vi "4-Build Do.vi"() -> ()   [LabVIEW 2014, in "TestVIs.lvlib"]
uses:
  TestVIs.lvlib
  <vilib>/Utility/traverseref.llb/TRef TravTarget.ctl
  <vilib>/Utility/miscctls.llb/LVPointTypeDef.ctl
  <vilib>/Utility/traverseref.llb/VI Scripting - Traverse.lvlib
  CSPP_Actor/CS++Actor.lvclass
panel:
  out "error out":errorcluster
  in  "error in (no error)":errorcluster
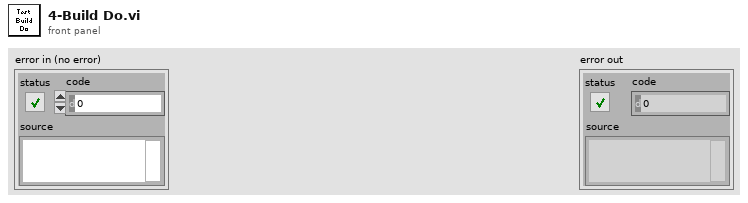
[diagram p1: front panel]
types:
  T1 = cluster{"Actor Method VI":refnum<vi>, "Actor Class":refnum<vi>, "Message Class":refnum<vi>}
  T2 = enum16{"Replace Class Controls/Constants", "Wire Special Inputs", "Wire Outputs", "Wire Method Inputs", "Connect Unbundler Input"}
  T3 = cluster{"Actor":cluster{"In":i32, "Out":i32}, "Error":cluster{"In":i32, "Out":i32}, "Terminals":cluster{"Position":enum16{"Left", "Top", "Bottom", "Right"}, "Terminal":i32}[]}
  T4 = typedef "TRef TravTarget.ctl" = enum16{"FP", "BD", "Other"}
  T5 = typedef "LVPointTypeDef.ctl" = cluster{"Horizontal":i16, "Vertical":i16}
  T6 = cluster{"Position":enum16{"Left", "Top", "Bottom", "Right"}, "Terminal":i32}[]
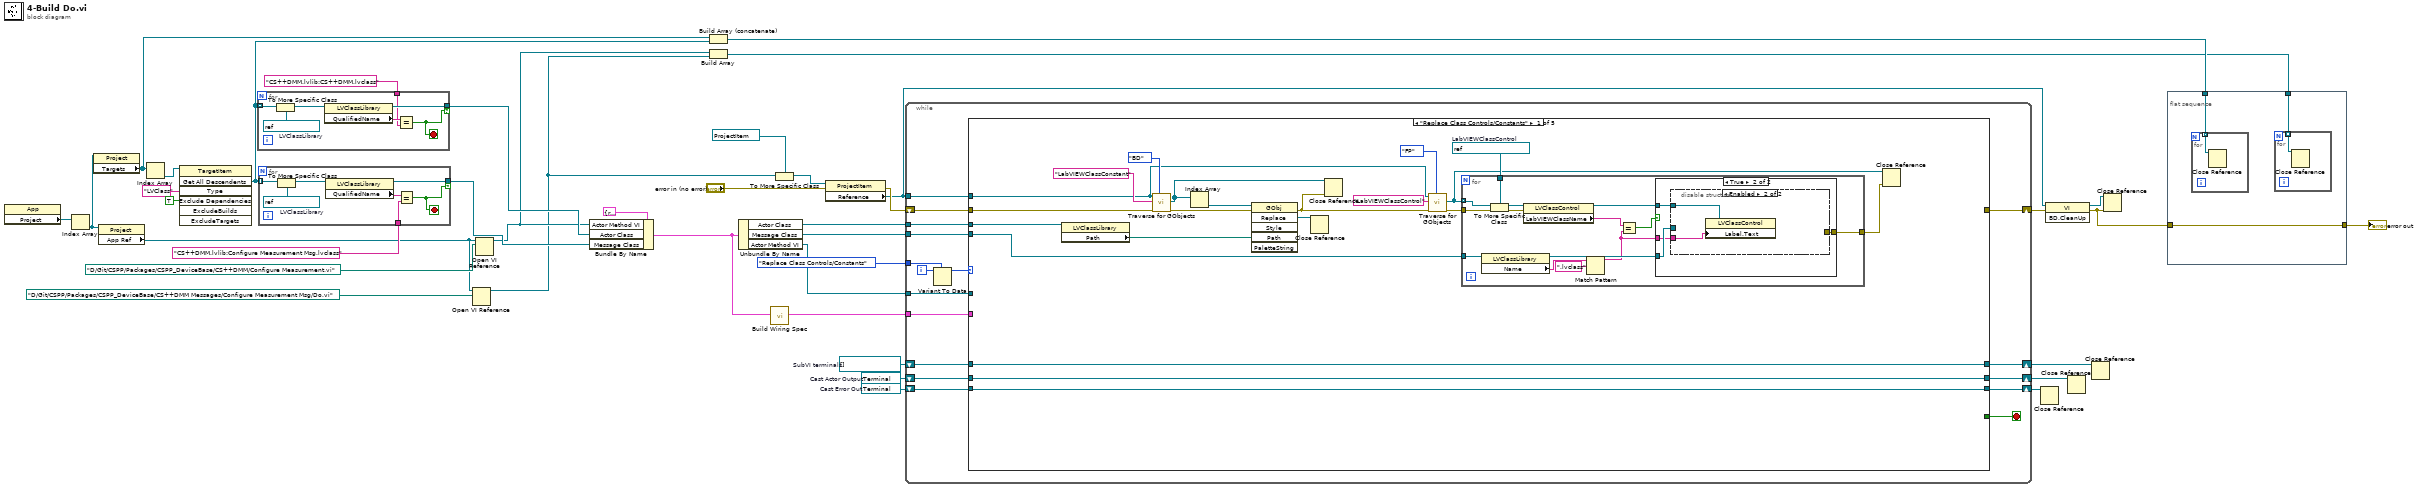
[diagram p0: block diagram]
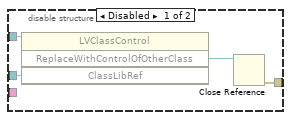
[diagram p3: hidden frame]
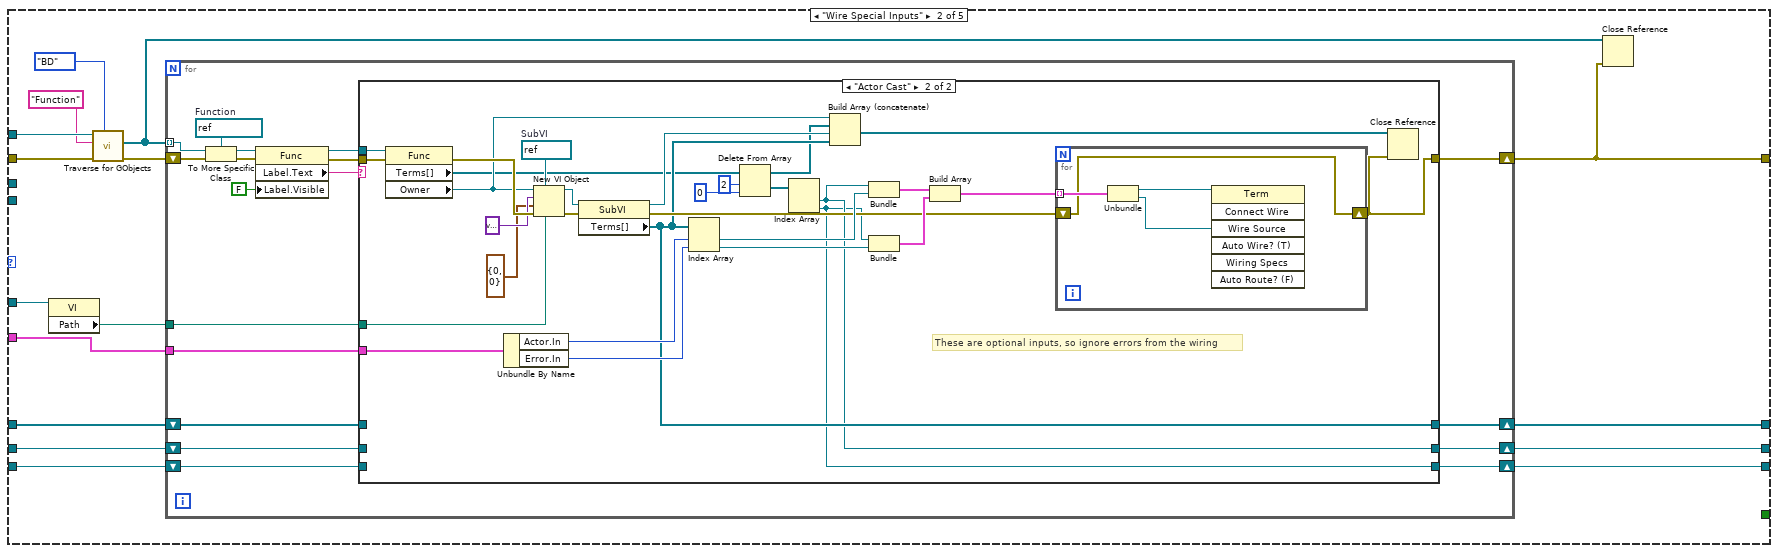
[diagram p4: hidden frame]
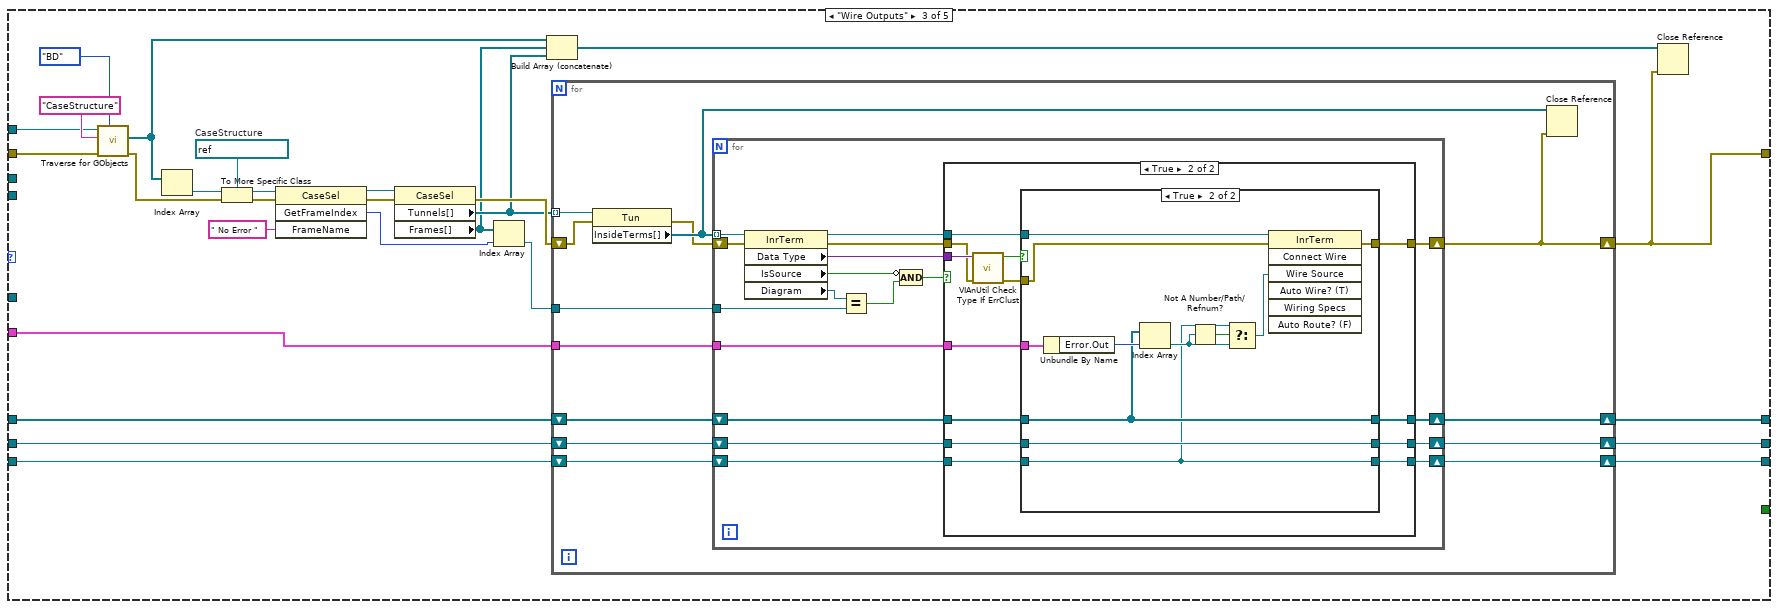
[diagram p6: hidden frame]
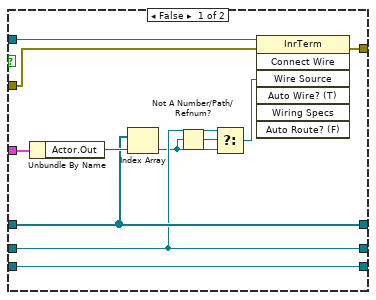
[diagram p8: hidden frame]
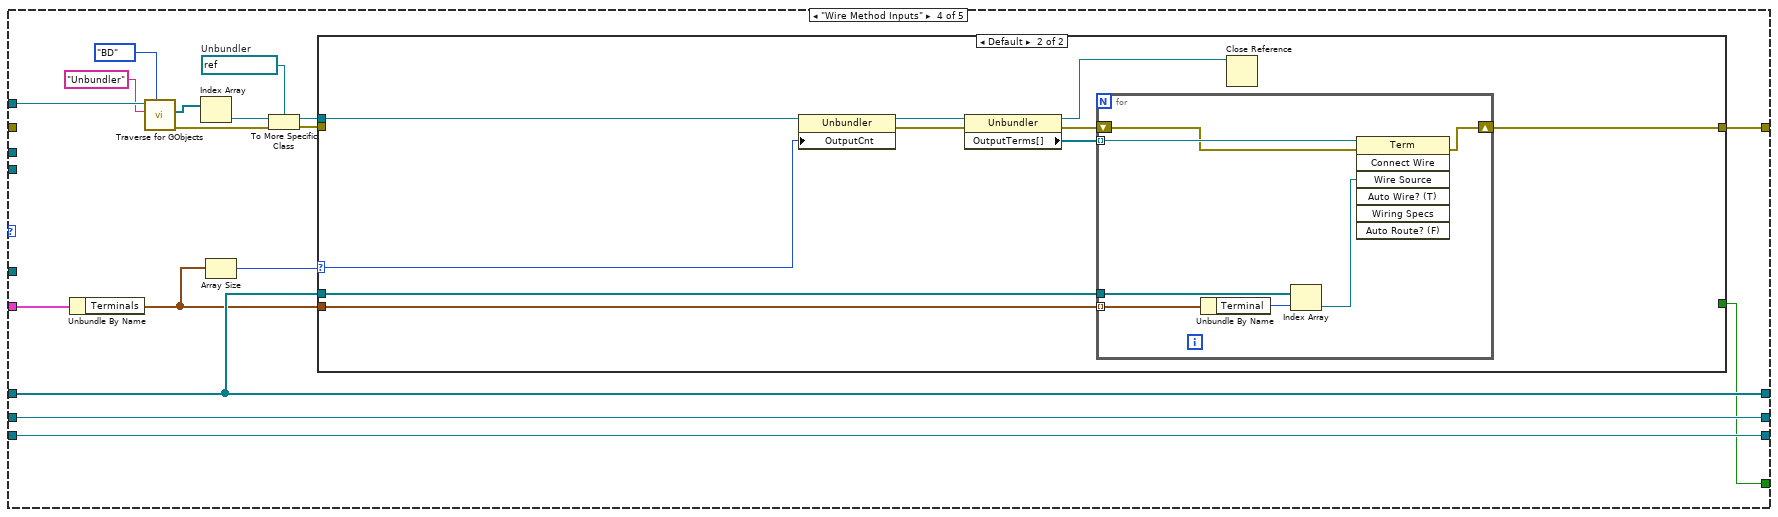
[diagram p9: hidden frame]
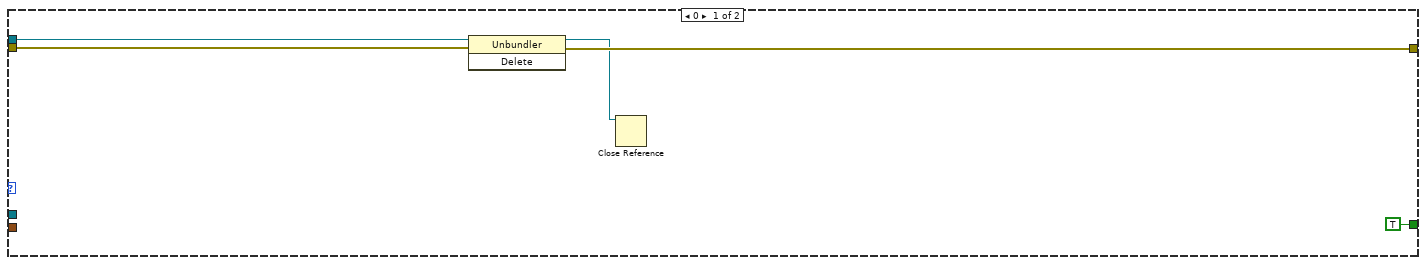
[diagram p10: hidden frame]
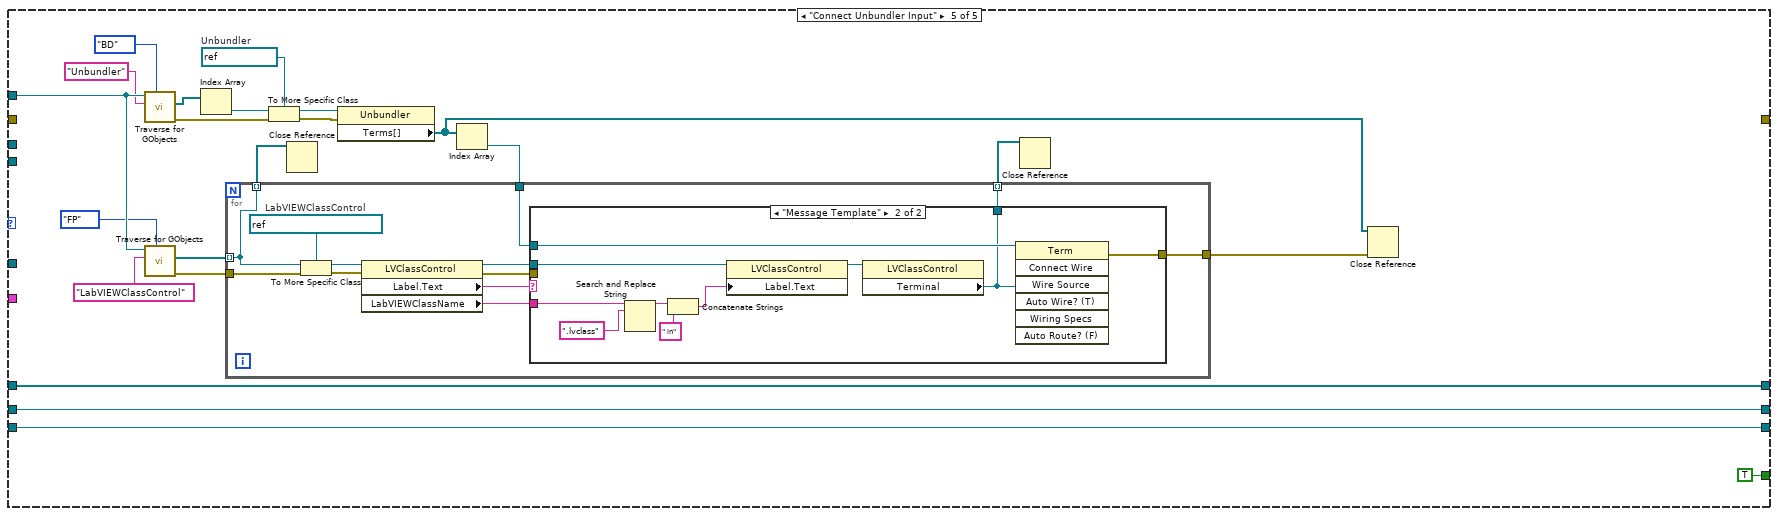
[diagram p11: hidden frame]
diagram:
  w31 = refnum<vi> refnum  # Cast Error Out
  w32 = refnum<vi> refnum  # Cast Actor Output
  w35 = refnum<vi>[] []  # SubVI terminals
  n1 = property class="App"() -> ("Project"=w24:refnum<vi>[])  [unwired: 2 in, 2 out]
  n2 = Index Array(array=w24) -> (element=w22:refnum<vi>)  [unwired: 1 in]
  n3 = property class="Project"(reference=w22) -> ("Targets"=w5:refnum<vi>[])  [unwired: 1 in, 2 out]
  n4 = property class="Project"(reference=w22) -> ("App Ref"=w16:refnum<vi>)  [unwired: 1 in, 2 out]
  n5 = Index Array(array=w5) -> (element=w21:refnum<vi>)  [unwired: 1 in]
  n6 = invoke class="TargetItem" method="Get All Descendents"(reference=w21, "Type"="LVClass", "Exclude Dependencies"=TRUE ("ExcludeDependencies")) -> ("All Descendents"=w6:refnum<vi>[])  [unwired: 4 in, 6 out]
  n7 = for {
    tunnel: [w44] -> w11 if=w42
    tunnel: w6 -> [w46] mode=indexing
    tunnel: "CS++DMM.lvlib:CS++DMM.lvclass" ("y") -> [w41]
    stop <- w42 stop-if-true
    w47 = refnum<vi> refnum  # LVClassLibrary
    n8 = To More Specific Class(target class=w47, reference=w46) -> (specific class reference=w45:refnum<vi>)  [unwired: 1 in, 1 out]
    n9 = property class="LVClassLibrary"(reference=w45) -> (reference out=w44:refnum<vi>, "QualifiedName"=w43:string)  [unwired: 1 in, 1 out]
    n10 = Equal?(x=w43, y=w41) -> (x = y?=w42:bool)
  }
  n11 = for {
    tunnel: [w51] -> w12 if=w48
    tunnel: w6 -> [w53] mode=indexing
    tunnel: "CS++DMM.lvlib:Configure Measurement Msg.lvclass" ("y") -> [w49]
    stop <- w48 stop-if-true
    w54 = refnum<vi> refnum  # LVClassLibrary
    n12 = To More Specific Class(target class=w54, reference=w53) -> (specific class reference=w52:refnum<vi>)  [unwired: 1 in, 1 out]
    n13 = property class="LVClassLibrary"(reference=w52) -> (reference out=w51:refnum<vi>, "QualifiedName"=w50:string)  [unwired: 1 in, 1 out]
    n14 = Equal?(x=w50, y=w49) -> (x = y?=w48:bool)
  }
  n15 = Open VI Reference(application reference (local)=w16, vi path=path "D:/Git/CSPP/Packages/CSPP_DeviceBase/CS++DMM Messages/Configure Measurement Msg/Do.vi") -> (vi reference=w3:refnum<vi>)  [unwired: 4 in, 1 out]
  n16 = Open VI Reference(application reference (local)=w16, vi path=path "D:/Git/CSPP/Packages/CSPP_DeviceBase/CS++DMM/Configure Measurement.vi") -> (vi reference=w4:refnum<vi>)  [unwired: 4 in, 1 out]
  n17 = Bundle By Name(cluster=T1 {"Actor Method VI"=refnum, "Actor Class"=refnum, "Message Class"=refnum} ("References"), "Actor Method VI"=w4, "Actor Class"=w11, "Message Class"=w12) -> (w10:T1)
  n18 = Build Array (concatenate)(w5, w6) -> (w2:refnum<vi>[])
  n19 = Build Array(w4, w3) -> (w1:refnum<vi>[])
  n20 = Unbundle By Name(w10) -> ("Actor Class"=w28:refnum<vi>, "Message Class"=w26:refnum<vi>, "Actor Method VI"=w27:refnum<vi>)
  n21 = call "Build Wiring Spec.vi"("References"=w10) -> ("Wiring Spec"=w25:T3)  [unwired: 9 in, 1 out]
  n22 = To More Specific Class(target class=refnum<vi> refnum ("Do VI"), reference=w3) -> (specific class reference=w14:refnum<vi>)  [unwired: 1 in, 1 out]
  n23 = property class="ProjectItem"(reference=w14, error in="error in (no error)") -> (error out=w40:errorcluster, "Reference"=w33:refnum<vi>)  [unwired: 1 out]
  n24 = while {
    tunnel: w33 -> [w71]
    tunnel: w25 -> [w69]
    shift-right: [w68] -> w38
    shift-left: w40 -> [w70]
    tunnel: T2."Replace Class Controls/Constants" -> [w66]
    tunnel: w28 -> [w64]
    tunnel: w27 -> [w63]
    shift-right: [w61] -> w34
    shift-left: w35 -> [w60]
    shift-right: [w59] -> w30
    shift-left: w32 -> [w57]
    shift-right: [w58] -> w29
    shift-left: w31 -> [w56]
    tunnel: w26 -> [w55]
    i -> [w67]
    stop <- w62 stop-if-true
    n25 = Variant To Data(type=w66, Variant=w67) -> (data=w65:T2)  [unwired: 1 in, 1 out]
    n26 = case shown="\"Replace Class Controls/Constants\"" w65 {
      tunnel: w71 -> [w79 w132 w213 w302 w346]
      tunnel: w70 -> [w86 w130 w212 _ _]
      tunnel: w69 -> [_ w128 w199 w295 _]
      tunnel: [_ w124 w197 w291 _] -> w68
      tunnel: w64 -> [w87 _ _ _ _]
      tunnel: w63 -> [_ w125 _ _ _]
      tunnel: [_ _ _ w286 TRUE] -> w62
      tunnel: [w83 w122 w200 w290 w345] -> w61
      tunnel: w60 -> [w83 w121 w201 w290 w345]
      tunnel: [w82 w120 w191 w289 w343] -> w59
      tunnel: [w81 w119 w189 w288 w342] -> w58
      tunnel: w57 -> [w82 w118 w192 w289 w343]
      tunnel: w56 -> [w81 w117 w190 w288 w342]
      tunnel: w55 -> [w74 _ _ _ _]
      frame "Replace Class Controls/Constants" {
        w77 = refnum<vi> refnum  # LabVIEWClassControl
        n27 = property class="LVClassLibrary"(reference=w87) -> ("Path"=w90:path)  [unwired: 1 in, 2 out]
        n28 = call <vilib>:"Traverse for GObjects.vi"("Traverse Target"=TRef_TravTarget."BD", "error in (no error)"=w86, "Class Name"="LabVIEWClassConstant", "VI Refnum"=w79) -> ("error out"=w91:errorcluster, "References"=w85:refnum<vi>[])  [unwired: 4 in, 2 out]
        n29 = Index Array(array=w85) -> (element=w89:refnum<vi>)  [unwired: 1 in]
        n30 = invoke class="GObj" method="Replace"(reference=w89, error in=w91, "Path"=w90) -> (error out=w80:errorcluster, "Replace"=w84:refnum<vi>)  [unwired: 3 in, 4 out]
        n31 = Close Reference(reference=w84) -> ()  [unwired: 1 in, 1 out]
        n32 = Close Reference(reference=w85, error in (no error)=w80) -> ()  [unwired: 1 out]
        n33 = call <vilib>:"Traverse for GObjects.vi"("Traverse Target"=TRef_TravTarget."FP", "error in (no error)"=w80, "Class Name"="LabVIEWClassControl", "VI Refnum"=w79) -> ("error out"=w75:errorcluster, "References"=w73:refnum<vi>[])  [unwired: 4 in, 2 out]
        n34 = for {
          tunnel: w77 -> [w106]
          tunnel: w75 -> [w105]
          tunnel: w73 -> [w104] mode=indexing
          tunnel: w74 -> [w99]
          tunnel: [w101] -> w72
          n35 = property class="LVClassLibrary"(reference=w99) -> (reference out=w98:refnum<vi>, "Name"=w95:string)  [unwired: 1 in, 1 out]
          n36 = To More Specific Class(target class=w106, reference=w104, error in=w105) -> (specific class reference=w100:refnum<vi>, error out=w102:errorcluster)
          n37 = property class="LVClassControl"(reference=w100, error in=w102) -> (reference out=w103:refnum<vi>, "LabVIEWClassName"=w97:string)  [unwired: 1 out]
          n38 = Match Pattern(string=w95, regular expression=".lvclass") -> (before substring=w94:string)  [unwired: 1 in, 3 out]
          n39 = Equal?(x=w97, y=w94) -> (x = y?=w96:bool)
          n40 = case shown="True" w96 {
            tunnel: w103 -> [_ w110]
            tunnel: w98 -> [_ w109]
            tunnel: [_ w108] -> w101
            tunnel: w94 -> [_ w107]
            frame False {
            }
            frame True {
              n41 = disable-structure shown="Enabled" {
                disable-tunnel: w110 -> [w114 w116]
                disable-tunnel: w109 -> [w113 _]
                disable-tunnel: [w111 _] -> w108
                disable-tunnel: w107 -> [_ w115]
                frame Disabled {
                  n42 = invoke class="LVClassControl" method="ReplaceWithControlOfOtherClass"(reference=w114, "ClassLibRef"=w113) -> ("ReplaceWithControlOfOtherClass"=w112:refnum<vi>)  [unwired: 2 in, 3 out]
                  n43 = Close Reference(reference=w112) -> (error out=w111:errorcluster)  [unwired: 1 in]
                }
                frame Enabled {
                  n44 = property class="LVClassControl"(reference=w116, "Label.Text"=w115) -> ()  [unwired: 1 in, 2 out]
                }
              }
            }
          }
        }
        n45 = Close Reference(reference=w73, error in (no error)=w72) -> ()  [unwired: 1 out]
      }
      frame "Wire Special Inputs" {
        n46 = property class="VI"(reference=w125) -> ("Path"=w126:path)  [unwired: 1 in, 2 out]
        n47 = call <vilib>:"Traverse for GObjects.vi"("Traverse Target"=TRef_TravTarget."BD", "error in (no error)"=w130, "Class Name"="Function", "VI Refnum"=w132) -> ("error out"=w129:errorcluster, "References"=w123:refnum<vi>[])  [unwired: 4 in, 2 out]
        n48 = for {
          tunnel: w123 -> [w148] mode=indexing
          tunnel: w126 -> [w143]
          tunnel: w128 -> [w141]
          shift-right: [w140] -> w124
          shift-left: w129 -> [w149]
          shift-right: [w138] -> w122
          shift-left: w121 -> [w137]
          shift-right: [w136] -> w120
          shift-left: w118 -> [w134]
          shift-right: [w135] -> w119
          shift-left: w117 -> [w133]
          w150 = refnum<vi> refnum  # Function
          n49 = To More Specific Class(target class=w150, reference=w148, error in=w149) -> (specific class reference=w147:refnum<vi>, error out=w146:errorcluster)
          n50 = property class="Func"(reference=w147, error in=w146, "Label.Visible"=FALSE) -> (reference out=w144:refnum<vi>, error out=w142:errorcluster, "Label.Text"=w145:string)
          n51 = case shown="\"Actor Cast\"" w145 {
            tunnel: w144 -> [_ w184]
            tunnel: w143 -> [_ w183]
            tunnel: w142 -> [w154 w181]
            tunnel: w141 -> [_ w176]
            tunnel: [w154 w165] -> w140
            tunnel: [w153 w162] -> w138
            tunnel: w137 -> [w153 _]
            tunnel: [w152 w156] -> w136
            tunnel: [w151 w155] -> w135
            tunnel: w134 -> [w152 _]
            tunnel: w133 -> [w151 _]
            frame Default {
            }
            frame "Actor Cast" {
              w182 = refnum<vi> refnum  # SubVI
              # "These are optional inputs, so ignore errors from the wiring"
              n52 = property class="Func"(reference=w184, error in=w181) -> (error out=w180:errorcluster, "Terms[]"=w161:refnum<vi>[], "Owner"=w163:refnum<vi>)  [unwired: 1 out]
              n53 = Unbundle By Name(w176) -> ("Actor.In"=w175:i32, "Error.In"=w174:i32)
              n54 = New VI Object(vi object class=w182, owner refnum=w163, style=variant, position/next to=T5 {"Horizontal"=0, "Vertical"=0} ("location"), 6:w183, 8:w180) -> (object refnum=w178:refnum<vi>, 0:w177:errorcluster)  [unwired: 2 in]
              n55 = property class="SubVI"(reference=w178, error in=w177) -> (reference out=w164:refnum<vi>, error out=w168:errorcluster, "Terms[]"=w162:refnum<vi>[])
              n56 = Index Array(array=w162, index #1=w175, index #2=w174) -> (element #1=w173:refnum<vi>, element #2=w172:refnum<vi>)
              n57 = Delete From Array(array=w161, length=2, index=0) -> (deleted portion=w157:refnum<vi>[], array with subset deleted=w159:refnum<vi>[])
              n58 = Index Array(array=w157) -> (element #1=w156:refnum<vi>, element #2=w155:refnum<vi>)  [unwired: 2 in]
              n59 = Build Array (concatenate)(w163, w159, w164, w162) -> (w166:refnum<vi>[])
              n60 = Bundle(w156, w173) -> (w171:cluster{refnum<vi>, refnum<vi>})  [unwired: 1 in]
              n61 = Bundle(w155, w172) -> (w170:cluster{refnum<vi>, refnum<vi>})  [unwired: 1 in]
              n62 = Build Array(w171, w170) -> (w169:cluster{refnum<vi>, refnum<vi>}[])
              n63 = for {
                tunnel: w169 -> [w188] mode=indexing
                shift-right: [w186] -> w165
                shift-left: w168 -> [w186]
                n64 = Unbundle(w188) -> (w187:refnum<vi>, w185:refnum<vi>)
                n65 = invoke class="Term" method="Connect Wire"(reference=w187, "Wire Source"=w185) -> ()  [unwired: 5 in, 7 out]
              }
              n66 = Close Reference(reference=w166, error in (no error)=w165) -> ()  [unwired: 1 out]
            }
          }
        }
        n67 = Close Reference(reference=w123, error in (no error)=w124) -> ()  [unwired: 1 out]
      }
      frame "Wire Outputs" {
        w210 = refnum<vi> refnum  # CaseStructure
        n68 = call <vilib>:"Traverse for GObjects.vi"("Traverse Target"=TRef_TravTarget."BD", "error in (no error)"=w212, "Class Name"="CaseStructure", "VI Refnum"=w213) -> ("error out"=w209:errorcluster, "References"=w193:refnum<vi>[])  [unwired: 4 in, 2 out]
        n69 = Index Array(array=w193) -> (element=w211:refnum<vi>)  [unwired: 1 in]
        n70 = To More Specific Class(target class=w210, reference=w211, error in=w209) -> (specific class reference=w206:refnum<vi>, error out=w205:errorcluster)
        n71 = invoke class="CaseSel" method="GetFrameIndex"(reference=w206, error in=w205, "FrameName"=" No Error " ("Frame Name")) -> (reference out=w207:refnum<vi>, error out=w208:errorcluster, "GetFrameIndex"=w203:i32)  [unwired: 1 in, 1 out]
        n72 = property class="CaseSel"(reference=w207, error in=w208) -> (error out=w198:errorcluster, "Tunnels[]"=w196:refnum<vi>[], "Frames[]"=w194:refnum<vi>[])  [unwired: 1 out]
        n73 = Index Array(array=w194, index=w203) -> (element=w202:refnum<vi>)
        n74 = Build Array (concatenate)(w193, w194, w196) -> (w195:refnum<vi>[])
        n75 = for {
          tunnel: w196 -> [w228] mode=indexing
          tunnel: w202 -> [w227]
          shift-right: [w225] -> w200
          shift-left: w201 -> [w226]
          tunnel: w199 -> [w224]
          shift-right: [w220] -> w197
          shift-left: w198 -> [w221]
          shift-right: [w218] -> w191
          shift-left: w192 -> [w219]
          shift-right: [w216] -> w189
          shift-left: w190 -> [w217]
          n76 = property class="Tun"(reference=w228, error in=w221) -> (error out=w222:errorcluster, "InsideTerms[]"=w223:refnum<vi>[])  [unwired: 1 out]
          n77 = for {
            tunnel: w223 -> [w246] mode=indexing
            tunnel: w227 -> [w244]
            shift-right: [w236] -> w225
            shift-left: w226 -> [w238]
            tunnel: w224 -> [w239]
            shift-right: [w234] -> w220
            shift-left: w222 -> [w233]
            shift-right: [w230] -> w218
            shift-left: w219 -> [w232]
            shift-right: [w229] -> w216
            shift-left: w217 -> [w231]
            n78 = property class="InrTerm"(reference=w246, error in=w233) -> (reference out=w237:refnum<vi>, error out=w235:errorcluster, "Data Type"=w240:variant, "IsSource"=w243:bool, "Diagram"=w245:refnum<vi>)
            n79 = Equal?(x=w245, y=w244) -> (x = y?=w242:bool)
            n80 = Compound Arithmetic op=AND(invert w243, w242) -> (w241:bool)
            n81 = case shown="True" w241 {
              tunnel: w240 -> [_ w263]
              tunnel: w239 -> [_ w261]
              tunnel: w238 -> [w250 w260]
              tunnel: w237 -> [_ w259]
              tunnel: [w250 w258] -> w236
              tunnel: w235 -> [w249 w255]
              tunnel: [w249 w257] -> w234
              tunnel: w232 -> [w248 w254]
              tunnel: w231 -> [w247 w253]
              tunnel: [w248 w252] -> w230
              tunnel: [w247 w251] -> w229
              frame False {
              }
              frame True {
                n82 = call <vilib>:"VIAnUtil Check Type If ErrClust.vi"("error in (no error)"=w255, "Data In"=w263) -> ("error out"=w256:errorcluster, "IsErrClust?"=w262:bool)  [unwired: 8 in]
                n83 = case shown="True" w262 {
                  tunnel: w261 -> [w274 w285]
                  tunnel: w260 -> [w271 w282]
                  tunnel: w259 -> [w272 w283]
                  tunnel: [w271 w282] -> w258
                  tunnel: [w270 w281] -> w257
                  tunnel: w256 -> [w269 w280]
                  tunnel: w254 -> [w267 w279]
                  tunnel: w253 -> [w268 w275]
                  tunnel: [w267 w279] -> w252
                  tunnel: [w268 w275] -> w251
                  frame False {
                    n84 = Unbundle By Name(w274) -> ("Actor.Out"=w273:i32)
                    n85 = Index Array(array=w271, index=w273) -> (element=w265:refnum<vi>)
                    n86 = Not A Number/Path/Refnum?(number/path/refnum=w265) -> (NaN/Path/Refnum?=w264:bool)
                    n87 = Select(t=w267, s=w264, f=w265) -> (s? t:f=w266:refnum<vi>)
                    n88 = invoke class="InrTerm" method="Connect Wire"(reference=w272, error in=w269, "Wire Source"=w266) -> (error out=w270:errorcluster)  [unwired: 4 in, 6 out]
                  }
                  frame True {
                    n89 = Unbundle By Name(w285) -> ("Error.Out"=w284:i32)
                    n90 = Index Array(array=w282, index=w284) -> (element=w277:refnum<vi>)
                    n91 = Not A Number/Path/Refnum?(number/path/refnum=w277) -> (NaN/Path/Refnum?=w276:bool)
                    n92 = Select(t=w275, s=w276, f=w277) -> (s? t:f=w278:refnum<vi>)
                    n93 = invoke class="InrTerm" method="Connect Wire"(reference=w283, error in=w280, "Wire Source"=w278) -> (error out=w281:errorcluster)  [unwired: 4 in, 6 out]
                  }
                }
              }
            }
          }
          n94 = Close Reference(reference=w223, error in (no error)=w220) -> ()  [unwired: 1 out]
        }
        n95 = Close Reference(reference=w195, error in (no error)=w197) -> ()  [unwired: 1 out]
      }
      frame "Wire Method Inputs" {
        w296 = refnum<vi> refnum  # Unbundler
        n96 = Unbundle By Name(w295) -> ("Terminals"=w287:T6)
        n97 = call <vilib>:"Traverse for GObjects.vi"("Traverse Target"=TRef_TravTarget."BD", "Class Name"="Unbundler", "VI Refnum"=w302) -> ("error out"=w297:errorcluster, "References"=w299:refnum<vi>[])  [unwired: 5 in, 2 out]
        n98 = Index Array(array=w299) -> (element=w298:refnum<vi>)  [unwired: 1 in]
        n99 = Array Size(array=w287) -> (size(s)=w294:i32)
        n100 = To More Specific Class(target class=w296, reference=w298, error in=w297) -> (specific class reference=w293:refnum<vi>, error out=w292:errorcluster)
        n101 = case shown="Default" w294 {
          selector: w294 -> [_ w312]
          tunnel: w293 -> [w307 w310]
          tunnel: w290 -> [_ w315]
          tunnel: w292 -> [w306 _]
          tunnel: [w305 w309] -> w291
          tunnel: w287 -> [_ w317]
          tunnel: [TRUE _] -> w286
          frame 0 {
            n102 = invoke class="Unbundler" method="Delete"(reference=w307, error in=w306) -> (reference out=w304:refnum<vi>, error out=w305:errorcluster)  [unwired: 1 in, 1 out]
            n103 = Close Reference(reference=w304) -> ()  [unwired: 1 in, 1 out]
          }
          frame Default {
            n104 = property class="Unbundler"(reference=w310, "OutputCnt"=w312) -> (reference out=w313:refnum<vi>, error out=w311:errorcluster)  [unwired: 1 in]
            n105 = property class="Unbundler"(reference=w313, error in=w311) -> (reference out=w308:refnum<vi>, error out=w314:errorcluster, "OutputTerms[]"=w316:refnum<vi>[])
            n106 = for {
              tunnel: w317 -> [w319] mode=indexing
              tunnel: w316 -> [w324] mode=indexing
              tunnel: w315 -> [w323]
              shift-right: [w320] -> w309
              shift-left: w314 -> [w321]
              n107 = Unbundle By Name(w319) -> ("Terminal"=w318:i32)
              n108 = Index Array(array=w323, index=w318) -> (element=w322:refnum<vi>)
              n109 = invoke class="Term" method="Connect Wire"(reference=w324, error in=w321, "Wire Source"=w322) -> (error out=w320:errorcluster)  [unwired: 4 in, 6 out]
            }
            n110 = Close Reference(reference=w308) -> ()  [unwired: 1 in, 1 out]
          }
        }
      }
      frame "Connect Unbundler Input" {
        w337 = refnum<vi> refnum  # Unbundler
        n111 = call <vilib>:"Traverse for GObjects.vi"("Traverse Target"=TRef_TravTarget."BD", "Class Name"="Unbundler", "VI Refnum"=w346) -> ("error out"=w338:errorcluster, "References"=w340:refnum<vi>[])  [unwired: 5 in, 2 out]
        n112 = call <vilib>:"Traverse for GObjects.vi"("Traverse Target"=TRef_TravTarget."FP", "Class Name"="LabVIEWClassControl", "VI Refnum"=w346) -> ("error out"=w336:errorcluster, "References"=w329:refnum<vi>[])  [unwired: 5 in, 2 out]
        n113 = Index Array(array=w340) -> (element=w339:refnum<vi>)  [unwired: 1 in]
        n114 = To More Specific Class(target class=w337, reference=w339, error in=w338) -> (specific class reference=w332:refnum<vi>, error out=w331:errorcluster)
        n115 = property class="Unbundler"(reference=w332, error in=w331) -> ("Terms[]"=w326:refnum<vi>[])  [unwired: 2 out]
        n116 = Index Array(array=w326) -> (element=w330:refnum<vi>)  [unwired: 1 in]
        n117 = for {
          tunnel: w336 -> [w358]
          tunnel: [w349] -> w333 mode=indexing
          tunnel: w330 -> [w351]
          tunnel: w329 -> [w349] mode=indexing
          tunnel: [w348] -> w327
          tunnel: [w347] -> w325 mode=indexing
          w357 = refnum<vi> refnum  # LabVIEWClassControl
          n118 = To More Specific Class(target class=w357, reference=w349, error in=w358) -> (specific class reference=w356:refnum<vi>, error out=w355:errorcluster)
          n119 = property class="LVClassControl"(reference=w356, error in=w355) -> (reference out=w353:refnum<vi>, error out=w352:errorcluster, "Label.Text"=w354:string, "LabVIEWClassName"=w350:string)
          n120 = case shown="\"Message Template\"" w354 {
            tunnel: w353 -> [_ w368]
            tunnel: w352 -> [_ _]
            tunnel: w351 -> [_ w367]
            tunnel: w350 -> [_ w363]
            tunnel: [_ w360] -> w348
            tunnel: [_ w359] -> w347
            frame Default {
            }
            frame "Message Template" {
              n121 = Search and Replace String(input string=w363, search string=".lvclass" ("regular expression")) -> (result string=w362:string)  [unwired: 6 in, 3 out]
              n122 = Concatenate Strings(w362, " in" ("string")) -> (w365:string)
              n123 = property class="LVClassControl"(reference=w368, "Label.Text"=w365) -> (reference out=w366:refnum<vi>)  [unwired: 1 in, 1 out]
              n124 = property class="LVClassControl"(reference=w366) -> ("Terminal"=w359:refnum<vi>)  [unwired: 1 in, 2 out]
              n125 = invoke class="Term" method="Connect Wire"(reference=w367, "Wire Source"=w359) -> (error out=w360:errorcluster)  [unwired: 5 in, 6 out]
            }
          }
        }
        n126 = Close Reference(reference=w333) -> ()  [unwired: 1 in, 1 out]
        n127 = Close Reference(reference=w325) -> ()  [unwired: 1 in, 1 out]
        n128 = Close Reference(reference=w326, error in (no error)=w327) -> ()  [unwired: 1 out]
      }
    }
  }
  n129 = Close Reference(reference=w29) -> ()  [unwired: 1 in, 1 out]
  n130 = invoke class="VI" method="BD.CleanUp"(reference=w33, error in=w38) -> (reference out=w37:refnum<vi>, error out=w7:errorcluster)  [unwired: 1 in, 1 out]
  n131 = Close Reference(reference=w30) -> ()  [unwired: 1 in, 1 out]
  n132 = Close Reference(reference=w34) -> ()  [unwired: 1 in, 1 out]
  n133 = Close Reference(reference=w37, error in (no error)=w7) -> ()  [unwired: 1 out]
  n134 = flat-sequence {
    tunnel: [w371] -> w8
    tunnel: w7 -> [w371]
    tunnel: w2 -> [w370]
    tunnel: w1 -> [w369]
    frame #0 {
      n135 = for {
        tunnel: w370 -> [w373] mode=indexing
        n136 = Close Reference(reference=w373) -> ()  [unwired: 1 in, 1 out]
      }
      n137 = for {
        tunnel: w369 -> [w372] mode=indexing
        n138 = Close Reference(reference=w372) -> ()  [unwired: 1 in, 1 out]
      }
    }
  }
  "error out" <- w8
